vi "Initialize.vi"(8 "Error In":errorcluster) -> (0 "Error Out":errorcluster, 3 "Dashboard":refnum<class "Dashboard.lvclass">)   [LabVIEW 2019, in "Dashboard.lvclass"]
uses:
  Dashboard.lvclass
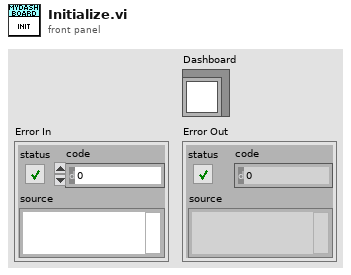
[diagram p1: front panel]
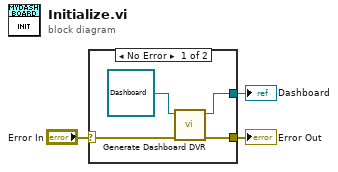
[diagram p0: block diagram]
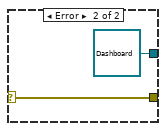
[diagram p2: hidden frame]
diagram:
  n1 = case shown="No Error" "Error In" {
    selector: "Error In" -> [w5 w9]
    tunnel: [w6 refnum<class "Dashboard.lvclass"> refnum ("Dashboard Out")] -> w3
    tunnel: [w4 w9] -> w1
    frame No Error {
      n2 = call "Generate Dashboard DVR.vi"("Error In"=w5, "Dashboard In"=refnum<class "Dashboard.lvclass"> refnum ("Dashboard")) -> ("Error Out"=w4:errorcluster, "Dashboard Out"=w6:refnum<class "Dashboard.lvclass">)  [unwired: 8 in]
    }
    frame Error {
    }
  }
  "Dashboard" <- w3
  "Error Out" <- w1
